vi "Data Logger Module.vi"(8 "Identifier":string, 11 "Message queue":refnum<queue>) -> ()   [LabVIEW 2018]
uses:
  Classes/Message/Message.lvclass
  Classes/Depth Data Message/Depth Data Message.lvclass
  Classes/Report File/Report File.lvclass
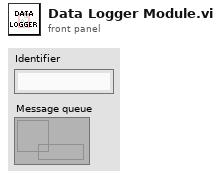
[diagram p1: front panel]
types:
  T1 = typedef "Roughness Parameters STYP.ctl" = cluster{"Normal":cluster{"Averages":cluster{"Average":dbl, "RMS":dbl, "Absolute Mean Deviation":dbl}, "Global Heuristics":cluster{"Max":dbl, "Min":dbl, "Max Peak-to-Peak":dbl}, "Skewdness":dbl, "Kurtosis":dbl, "RzDIN":dbl, "RzJIS":dbl}, "Slope Parameters":cluster{"Rdq":dbl, "Rda":dbl}, "Areal Roughness":cluster{"Peak Density":dbl}}
  T2 = cluster{"Normal":cluster{"Averages":cluster{"Average":dbl, "RMS":dbl, "Absolute Mean Deviation":dbl}, "Global Heuristics":cluster{"Max":dbl, "Min":dbl, "Max Peak-to-Peak":dbl}, "Skewdness":dbl, "Kurtosis":dbl, "RzDIN":dbl, "RzJIS":dbl}, "Slope Parameters":cluster{"Rdq":dbl, "Rda":dbl}, "Areal Roughness":cluster{"Peak Density":dbl}}
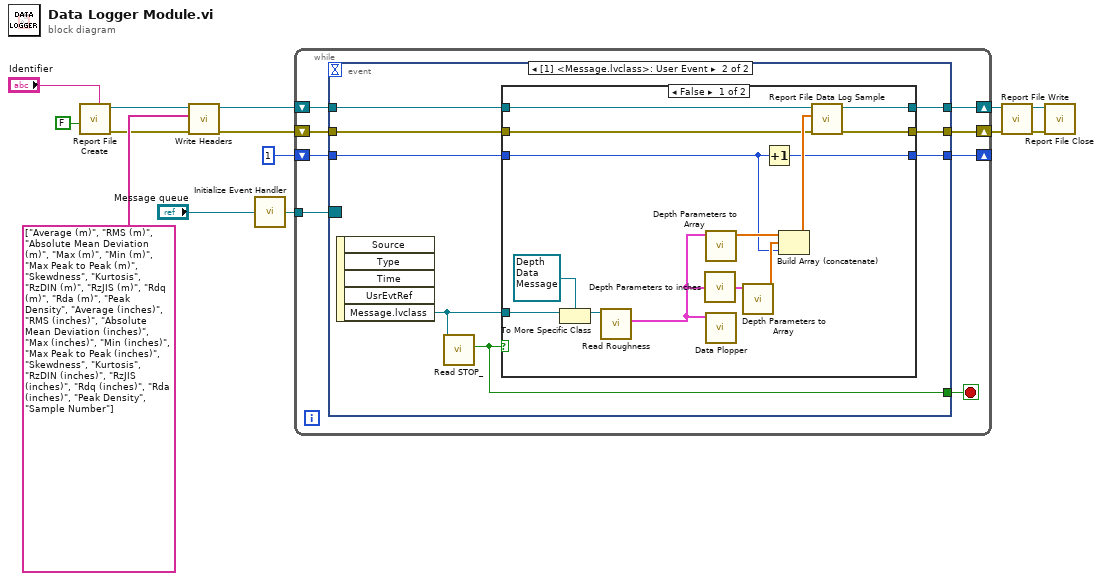
[diagram p0: block diagram]
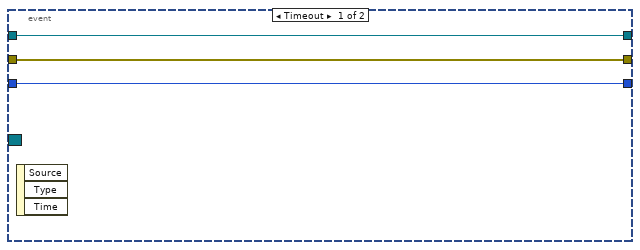
[diagram p2: hidden frame]
diagram:
  n1 = call "Report File Create.vi"("Identifier (\"\")"="Identifier", "Open? (T)"=FALSE) -> ("error out"=w11:errorcluster, "Report File out"=w13:refnum<class "Report File.lvclass">)  [unwired: 8 in]
  n2 = call-dynamic "Write Headers.vi"("error in (no error)"=w11, "Headers"=string[] ["Average (m)", "RMS (m)", "Absolute Mean Deviation (m)", "Max (m)", "Min (m)", "Max Peak to Peak (m)", "Skewdness", "Kurtosis", "RzDIN (m)", "RzJIS (m)", "Rdq (m)", "Rda (m)", "Peak Density", "Average (inches)", "RMS (inches)", "Absolute Mean Deviation (inches)", "Max (inches)", "Min (inches)", "Max Peak to Peak (inches)", "Skewdness", "Kurtosis", "RzDIN (inches)", "RzJIS (inches)", "Rdq (inches)", "Rda (inches)", "Peak Density", "Sample Number"], "Report File in"=w13) -> ("error out"=w4:errorcluster, "Report File out"=w5:refnum<class "Report File.lvclass">)  [unwired: 7 in]
  n3 = call "Initialize Event Handler.vi"("data queue"="Message queue") -> ("Event Refnum"=w6:refnum<event-registration>)
  n4 = while {
    tunnel: w6 -> [w22]
    shift-right: [w18] -> w2
    shift-left: w5 -> [w20]
    shift-right: [w17] -> w1
    shift-left: w4 -> [w19]
    shift-right: [w15] -> _
    shift-left: 1 -> [w16]
    stop <- w21 stop-if-true
    n5 = event shown="[1] <Message.lvclass>: User Event" {
      selector: w22 -> [_ _]
      dyn-events: _ -> [_ _]
      timeout: _ -> [_ _]
      tunnel: [_ w33] -> w21
      tunnel: w20 -> [w25 w31]
      tunnel: w19 -> [w24 w30]
      tunnel: [w25 w29] -> w18
      tunnel: [w24 w28] -> w17
      tunnel: w16 -> [w23 w27]
      tunnel: [w23 w26] -> w15
      event Timeout {
        n6 = event-data() -> ()  [unwired: 1 in, 3 out]
      }
      event User Event {
        n7 = event-data() -> ("Message.lvclass"=w32:refnum<class "Message.lvclass">)  [unwired: 1 in, 4 out]
        n8 = call-dynamic "Read STOP_.vi"("Message in"=w32) -> ("STOP?"=w33:bool)  [unwired: 8 in, 2 out]
        n9 = case shown="False" w33 {
          tunnel: w32 -> [w47 _]
          tunnel: w31 -> [w39 w50]
          tunnel: w30 -> [w38 w49]
          tunnel: [w37 w50] -> w29
          tunnel: [w36 w49] -> w28
          tunnel: w27 -> [w35 w48]
          tunnel: [w34 w48] -> w26
          frame False {
            n10 = To More Specific Class(target class=refnum<class "Depth Data Message.lvclass"> refnum ("Depth Data Message.lvclass"), reference=w47) -> (specific class reference=w45:refnum<class "Depth Data Message.lvclass">)  [unwired: 1 in, 1 out]
            n11 = call-dynamic "Read Roughness.vi"("Depth Data Message in"=w45) -> ("Roughness"=w40:T1)  [unwired: 8 in, 2 out]
            n12 = call "Depth Parameters to inches.vi"("Roughness Parameters"=w40) -> ("Roughness Parameters (inches)"=w44:T2)
            n13 = call "Depth Parameters to Array.vi"("Roughness Parameters in"=w40) -> ("Array"=w43:dbl[])  [unwired: 10 in]
            n14 = call "Data Plopper.vi"("Roughness"=w40) -> ()  [unwired: 11 in]
            n15 = call "Depth Parameters to Array.vi"("Roughness Parameters in"=w44) -> ("Array"=w42:dbl[])  [unwired: 10 in]
            n16 = Increment(x=w35) -> (x+1=w34:i32)
            n17 = Build Array (concatenate)(w43, w42, w35) -> (w41:dbl[])
            n18 = call-dynamic "Report File Data Log Sample.vi"("error in (no error)"=w38, "Data Row"=w41, "Report File in"=w39) -> ("error out"=w36:errorcluster, "Report File out"=w37:refnum<class "Report File.lvclass">)  [unwired: 7 in]
          }
          frame True {
          }
        }
      }
    }
  }
  n19 = call-dynamic "Report File Write.vi"("error in (no error)"=w1, "Report File in"=w2) -> ("error out"=w9:errorcluster, "Report File out"=w10:refnum<class "Report File.lvclass">)  [unwired: 8 in]
  n20 = call-dynamic "Report File Close.vi"("error in (no error)"=w9, "Report File in"=w10) -> ()  [unwired: 8 in, 2 out]
